vi "Init.vi"(8 "error in":errorcluster, 10 "OD Entry":refnum<class "OD Entry.lvclass">, 11 "RX COM PAM in":refnum<class "RX PDO Communication Parameter.lvclass">) -> (0 "error out":errorcluster, 3 "RX COM PAM out":refnum<class "RX PDO Communication Parameter.lvclass">)   [LabVIEW 2020, in "PDO Grid.lvlib" / "RX PDO Communication Parameter.lvclass"]
uses:
  RX PDO Communication Parameter.lvclass
  RX PDO Communication Parameter.lvclass/RX PDO Communication Parameter.ctl
  Core/OD Entry/OD Entry.lvclass
  Core/Value/Value.lvclass
  Core/PDO Communication Parameter/PDO Communication Parameter.lvclass
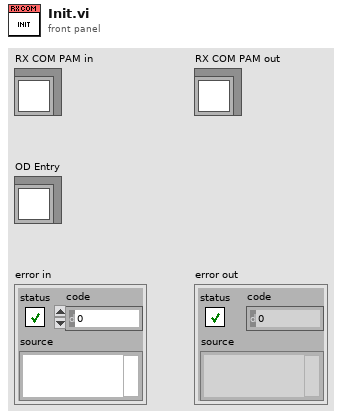
[diagram p1: front panel]
types:
  T1 = enum16{"ro", "wo", "rw", "rwr", "rww", "const", "UNKNOWN"}
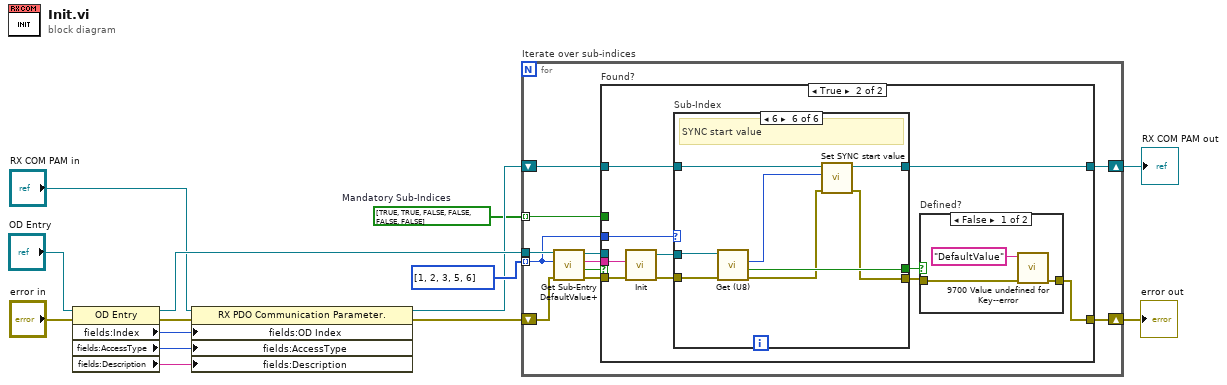
[diagram p0: block diagram]
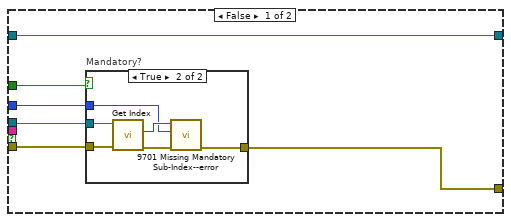
[diagram p2: hidden frame]
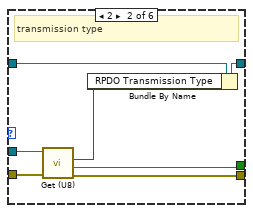
[diagram p5: hidden frame]
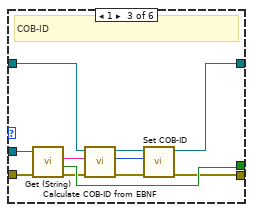
[diagram p6: hidden frame]
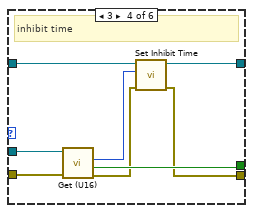
[diagram p7: hidden frame]
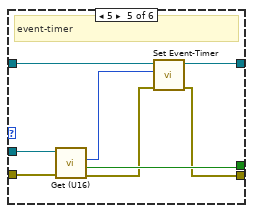
[diagram p8: hidden frame]
diagram:
  w1 = bool[] [TRUE, TRUE, FALSE, FALSE, FALSE, FALSE]  # Mandatory Sub-Indices
  n1 = property class="OD Entry"(reference="OD Entry", error in="error in") -> (reference out=w8:refnum<class "OD Entry.lvclass">, error out=w10:errorcluster, "fields:Index"=w5:u16, "fields:AccessType"=w4:T1, "fields:Description"=w3:string)
  n2 = property class="RX PDO Communication Parameter."(reference="RX COM PAM in", error in=w10, "fields:OD Index"=w5, "fields:AccessType"=w4, "fields:Description"=w3) -> (reference out=w6:refnum<class "RX PDO Communication Parameter.lvclass">, error out=w7:errorcluster)
  n3 = for "Iterate over sub-indices" {
    tunnel: u16[] [1, 2, 3, 5, 6] -> [w20] mode=indexing
    shift-right: [w24] -> w11
    shift-left: w6 -> [w25]
    shift-right: [w23] -> w12
    shift-left: w7 -> [w19]
    tunnel: w8 -> [w22]
    tunnel: w1 -> [w15] mode=indexing
    n4 = call "Get Sub-Entry DefaultValue+.vi"("Error In"=w19, "Sub-Index"=w20, "reference in"=w22) -> ("Error Out"=w18:errorcluster, "Found?"=w17:bool, "DefaultValue"=w16:string, "reference out"=w21:refnum<class "OD Entry.lvclass">)  [unwired: 5 in]
    n5 = case "Found?" shown="True" w17 {
      tunnel: w25 -> [w27 w48]
      tunnel: [w27 w47] -> w24
      tunnel: [w28 w40] -> w23
      tunnel: w21 -> [w30 _]
      tunnel: w20 -> [w29 w46]
      tunnel: w18 -> [w31 w45]
      tunnel: w16 -> [_ w39]
      tunnel: w15 -> [w26 _]
      frame False {
        n6 = case "Mandatory?" shown="True" w26 {
          tunnel: w31 -> [w32 w37]
          tunnel: w30 -> [_ w36]
          tunnel: w29 -> [_ w33]
          tunnel: [w32 w35] -> w28
          frame False {
          }
          frame True {
            n7 = call "Get Index.vi"("Error In"=w37, "reference in"=w36) -> ("Error Out"=w38:errorcluster, "Index"=w34:u16)  [unwired: 7 in, 1 out]
            n8 = call "9701 Missing Mandatory Sub-Index--error.vi"("error in"=w38, "Sub-Index"=w33, "Index"=w34) -> ("error out"=w35:errorcluster)  [unwired: 8 in]
          }
        }
      }
      frame True {
        n9 = call "Init.vi"("error in"=w45, "Value"=w39) -> ("error out"=w44:errorcluster, "Value out"=w43:refnum<class "Value.lvclass">)  [unwired: 8 in]
        n10 = case "Sub-Index" shown="6" w46 {
          tunnel: w48 -> [w50 w57 w63 w72 w83 w88]
          tunnel: [w50 w56 w59 w71 w79 w87] -> w47
          tunnel: w44 -> [w49 w54 w65 w74 w82 w91]
          tunnel: w43 -> [_ w53 w67 w75 w81 w90]
          tunnel: [_ w52 w66 w73 w80 w89] -> w42
          tunnel: [w49 w51 w61 w68 w77 w84] -> w41
          frame Default {
            # "can't be reached"
          }
          frame 2 {
            # "transmission type"
            n11 = call "Get (U8).vi"("error in"=w54, "Value in"=w53) -> ("error out"=w51:errorcluster, "Defined?"=w52:bool, "Value"=w55:u8)  [unwired: 6 in, 1 out]
            n12 = Bundle By Name(cluster=w57, "RPDO Transmission Type"=w55) -> (w56:refnum<class "RX PDO Communication Parameter.lvclass">)
          }
          frame 1 {
            # "COB-ID"
            n13 = call "Get (String).vi"("Value in"=w67) -> ("Defined?"=w66:bool, "Value"=w64:string)  [unwired: 8 in, 1 out]
            n14 = call "Calculate COB-ID from EBNF.vi"("error in"=w65, "ENBF"=w64, "Transmit PDO in"=w63) -> ("error out"=w62:errorcluster, "COB-ID"=w58:u32, "Transmit PDO out"=w60:refnum<class "RX PDO Communication Parameter.lvclass">)  [unwired: 6 in]
            n15 = call "Set COB-ID.vi"("error in (no error)"=w62, "COB-ID"=w58, "PDO Communication Parameter in"=w60) -> ("error out"=w61:errorcluster, "PDO Communication Parameter out"=w59:refnum<class "RX PDO Communication Parameter.lvclass">)  [unwired: 7 in]
          }
          frame 3 {
            # "inhibit time"
            n16 = call "Get (U16).vi"("error in"=w74, "Value in"=w75) -> ("error out"=w69:errorcluster, "Defined?"=w73:bool, "Value"=w70:u16)  [unwired: 6 in, 1 out]
            n17 = call "Set Inhibit Time.vi"("error in"=w69, "Inhibit Time"=w70, "PDO Communication Parameter in"=w72) -> ("error out"=w68:errorcluster, "PDO Communication Parameter out"=w71:refnum<class "RX PDO Communication Parameter.lvclass">)  [unwired: 7 in]
          }
          frame 5 {
            # "event-timer"
            n18 = call "Get (U16).vi"("error in"=w82, "Value in"=w81) -> ("error out"=w78:errorcluster, "Defined?"=w80:bool, "Value"=w76:u16)  [unwired: 6 in, 1 out]
            n19 = call "Set Event-Timer.vi"("error in (no error)"=w78, "Event-Timer"=w76, "PDO Communication Parameter in"=w83) -> ("error out"=w77:errorcluster, "PDO Communication Parameter out"=w79:refnum<class "RX PDO Communication Parameter.lvclass">)  [unwired: 7 in]
          }
          frame 6 {
            # "SYNC start value"
            n20 = call "Get (U8).vi"("error in"=w91, "Value in"=w90) -> ("error out"=w85:errorcluster, "Defined?"=w89:bool, "Value"=w86:u8)  [unwired: 6 in, 1 out]
            n21 = call "Set SYNC start value.vi"("error in (no error)"=w85, "SYNC start value"=w86, "PDO Communication Parameter in"=w88) -> ("error out"=w84:errorcluster, "PDO Communication Parameter out"=w87:refnum<class "RX PDO Communication Parameter.lvclass">)  [unwired: 7 in]
          }
        }
        n22 = case "Defined?" shown="False" w42 {
          tunnel: w41 -> [w94 w95]
          tunnel: [w92 w95] -> w40
          frame False {
            n23 = call "9700 Value undefined for Key--error.vi"("error in"=w94, "Argument"="DefaultValue" ("key")) -> ("error out"=w92:errorcluster)  [unwired: 9 in]
          }
          frame True {
          }
        }
      }
    }
  }
  "RX COM PAM out" <- w11
  "error out" <- w12
